vi "for_autoindexado.vi"() -> ()   [LabVIEW 2020]
panel:
  out "Array 2":dbl[](array[numeric])
  out "Array":i32[](array[numeric])
  out "Thermometer":dbl(slide) scale=0.0..100.0
  out "Iteraciones":i32
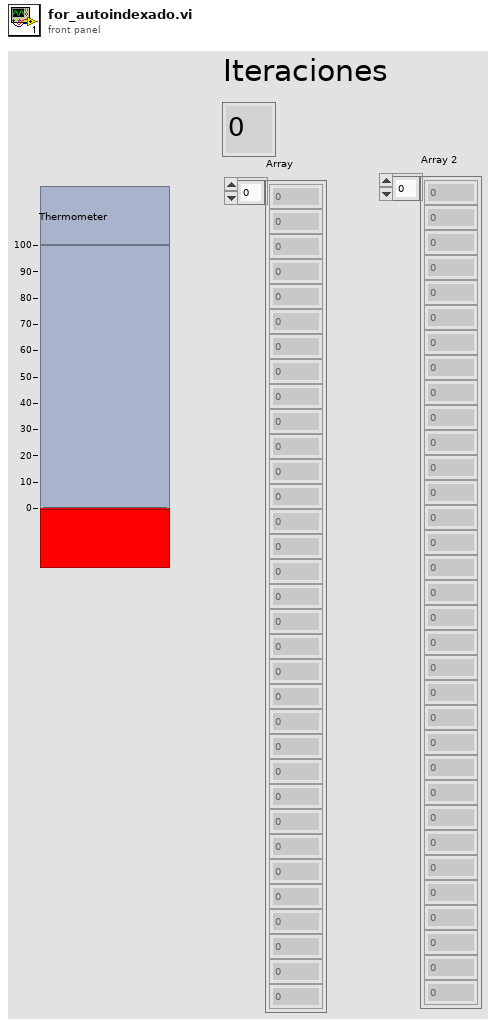
[diagram p1: front panel]
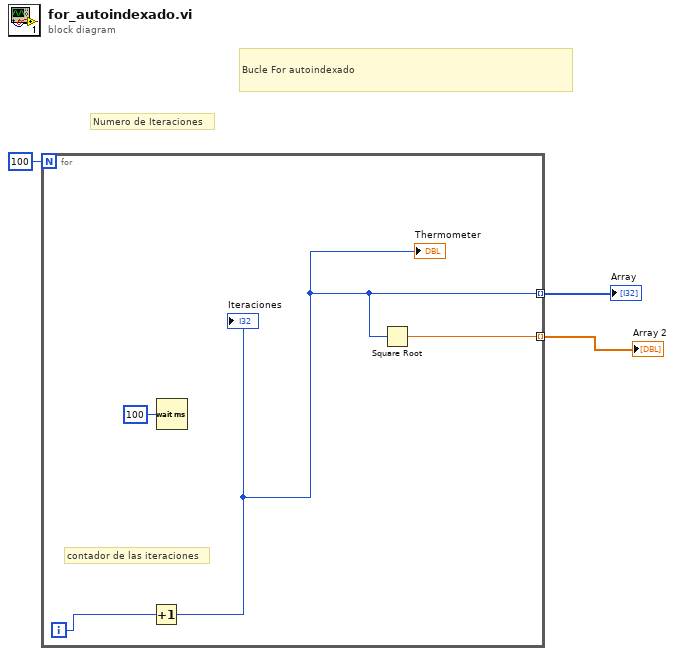
[diagram p0: block diagram]
diagram:
  # "Bucle For autoindexado"
  # "Numero de Iteraciones"
  n1 = for {
    N: 100 -> [_]
    tunnel: [w5] -> w2 mode=indexing
    tunnel: [w4] -> w1 mode=indexing
    i -> [w6]
    # "contador de las iteraciones"
    n2 = Increment(x=w6) -> (x+1=w5:i32)
    "Iteraciones" <- w5
    "Thermometer" <- w5
    n3 = Wait (ms)(milliseconds to wait=u32 100) -> ()  [unwired: 1 out]
    n4 = Square Root(x=w5) -> (sqrt(x)=w4:dbl)
  }
  "Array" <- w2
  "Array 2" <- w1
